vi "PrefDialog.vi"(8 "error in (no error)":errorcluster, 11 "ChromaPowerSupplyModel in":refnum<class "ChromaPowerSupplyModel.lvclass">) -> (0 "error out":errorcluster, 1 "Save As":bool, 2 "Changed":bool, 3 "MyPluginsBase out":refnum<class "ChromaPowerSupplyModel.lvclass">)   [LabVIEW 2018, in "AcPwrPlugins.lvlib" / "ChromaPowerSupplyModel.lvclass"]
doc: "This VI displays the prior instruments properties and allows a user to change the instrument properties and save these new set properties to the same location on disk or in a new location with a new name called \"Type\"."
uses:
  ChromaPowerSupplyModel.lvclass
  C:/Program Files (x86)/National Instruments/LabVIEW 2018/user.lib/NIST/BaseClasses/BasePlugin_class/BasePlugin.lvclass
  C:/Projects/SmartGrid/ICDAS/NistPluggableModules/AcPwr/AcPwrPlugins/AcPwrBaseClass/AcPwrBase.lvclass
  ChromaPowerSupplyClass/TypeDefs/Measurements.ctl
  AcPwrBaseClass/TypeDefs/BaseMeasurements.ctl
  ChromaAcLoadClass/TypeDefs/MeasurementType.ctl
  ChromaPowerSupplyClass/TypeDefs/Device(s)Settings.ctl
  TypeDefs/Database Settings.ctl
  <userlib>/NIST/BaseClasses/BasePlugin_class/BasePlugin.lvclass/BasePlugin.ctl
  AcPwrBaseClass/AcPwrBase.lvclass/AcPwrBase.ctl
  <userlib>/NIST/BaseClasses/BasePlugin_class/Accessors/Read PluginIniFilePath.vi
  AcPwrBaseClass/Accessors/Read BaseConfig.vi
  AcPwrBaseClass/Accessors/Read BaseMeasurements.vi
  <userlib>/NIST/BaseClasses/BasePlugin_class/Accessors/Write PluginIniFilePath.vi
  <vilib>/Utility/config.llb/NI_LVConfig.lvlib
  AcPwrBaseClass/AcPwrBase.lvclass
  ChromaPowerSupplyClass/ChromaPowerSupply.lvclass
  ChromaAcLoadClass/ChromaAcLoad.lvclass
panel:
  in  "Database Settings":T1
  in  "btnSaveAs":bool
  in  "btnSave":bool
  in  "Measurement RefreshTime (ms)":u32
  in  "Device(s)Settings":T2
  in  "BaseMeasurements":T3 {"NHRGridSim Phase" items=["All", "A Phase", "B Phase", "C Phase"]; "NHRDC Measurement Type" items=["Voltage"=1, "Positive Peak Voltage"=2, "Positive Peak Voltage Last Fetch"=4, "Negative Peak Voltage"=8, "Negative Peak Voltage Last Fetch"=16, "Current"=32, "Positive Peak Current"=64, "Positive Peak Current Last Fetch"=128, "Negative Peak Current"=256, "Negative Peak Current Last Fetch"=512, "Power"=1024, "Positive Peak Power"=2048, "Positive Peak Power Last Fetch"=4096, "Negative Peak Power"=8192, "Negative Peak Power Last Fetch"=16384, "Timestamp"=32768, "Charge Time"=65536, "Discharge Time"=131072, "Amp Hour"=262144, "Amp Hour Time"=524288, "Amp Hour Charge"=1048576, "Amp Hour Discharge"=2097152, "Kilo Watt Hour"=4194304, "Kilo Watt Hour Time"=8388608, "Kilo Watt Hour Charge"=16777216, "Kilo Watt Hour Discharge"=33554432, "UUT Temperature"=67108864]; "NHRDC Fetch Method" items=["Aperture", "Immediate"]}
  in  "Measurements":T5
  in  "btnCancel":bool
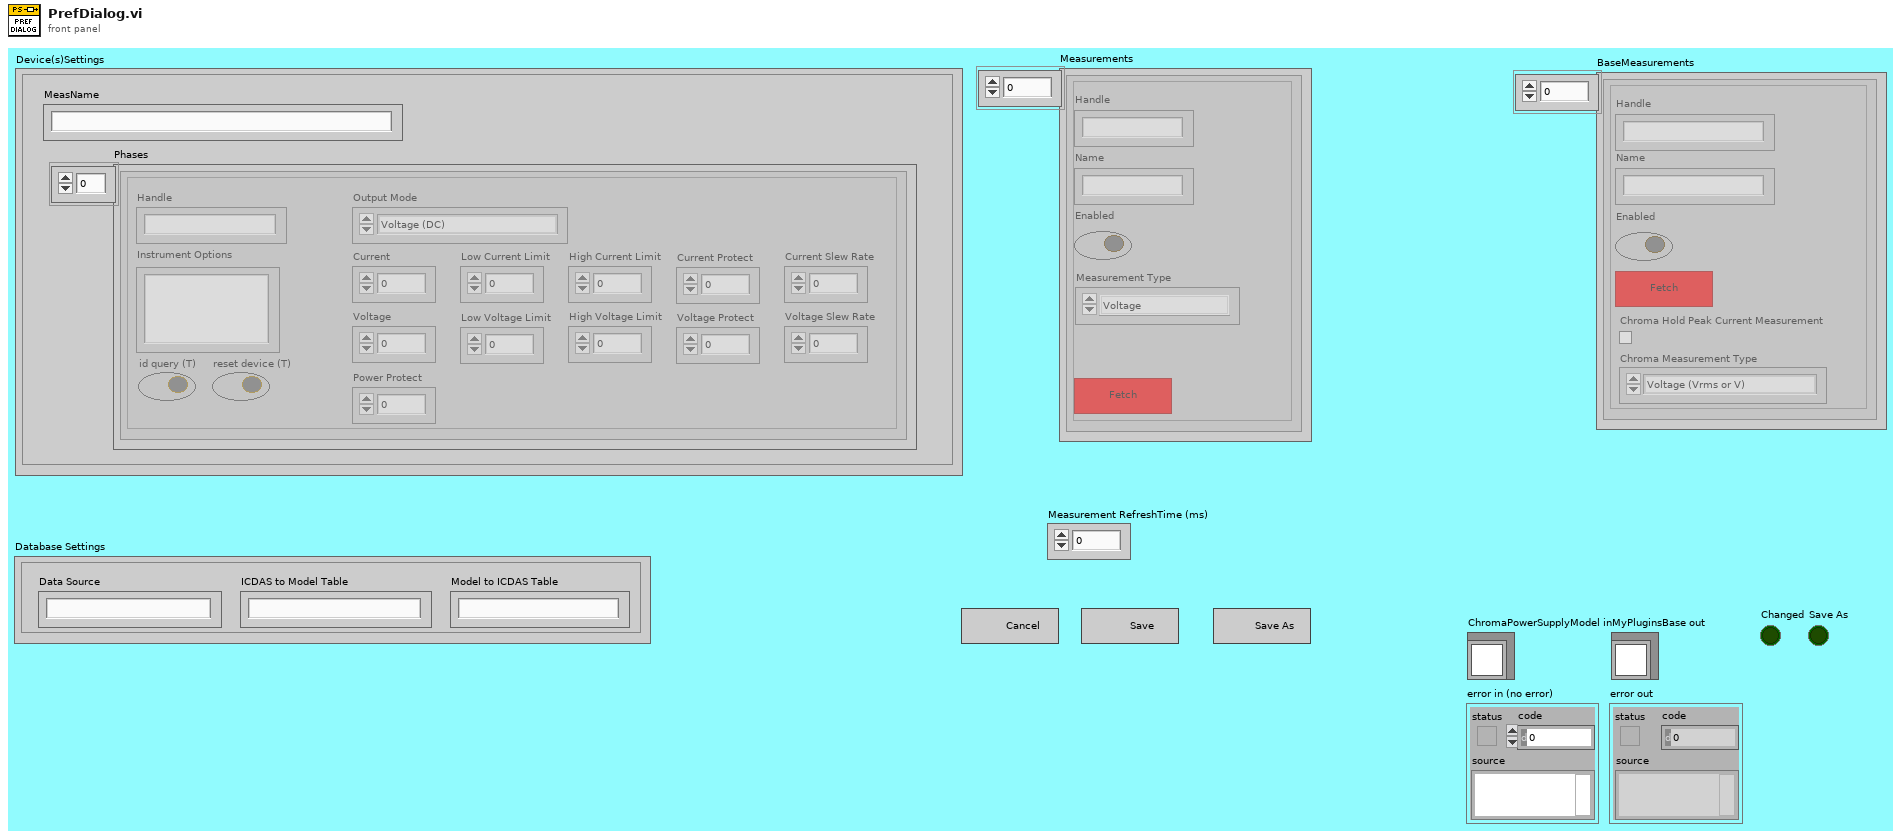
[diagram p1: front panel]
types:
  T1 = typedef "AcPwrPlugins.lvlib/ChromaPowerSupplyModel.lvclass/Database Settings.ctl" = cluster{"Data Source":string, "ICDAS to Model Table":string, "Model to ICDAS Table":string}
  T2 = typedef "AcPwrPlugins.lvlib/ChromaPowerSupply.lvclass/Device(s)Settings.ctl" = cluster{"Phases":cluster{"Handle":string, "Instrument Options":string, "id query (T)":bool, "reset device (T)":bool, "Timing":cluster{"TimingOn":enum16{""}, "Hours":u32, "Minutes":u32, "Seconds":dbl, "CutoffVoltage":dbl}, "Connected":bool, "Output Mode":enum16{"Voltage (DC)", "Current (DC)"}, "Voltage":dbl, "Current":dbl, "High Voltage Limit":dbl, "High Current Limit":dbl, "Power Protect":dbl, "Current Protect":dbl, "Voltage Protect":dbl, "Low Current Limit":dbl, "Low Voltage Limit":dbl, "Current Slew Rate":dbl, "Voltage Slew Rate":dbl}[], "MeasName":string}
  T3 = typedef "AcPwrPlugins.lvlib/AcPwrBase.lvclass/BaseMeasurements.ctl" = cluster{"Handle":string, "Name":string, "Enabled":bool, "Measurement Value":dbl, "btnMeasFetch":bool, "Chroma Hold Peak Current Measurement":bool, "Chroma Measurement Type":T4, "Chroma Protection Status String":string, "NHRDC Fetch Method":i32, "NHRDC Fetch Time (s)":sgl, "NHRDC Measurement Type":i32, "NHRGridSim Measurement Type ":enum16{"Average Current", "Max Current", "Min Current", "Average Voltage", "Max Voltage", "Min Voltage", "Average True Power", "Max True Power", "Min True Power", "Average Apparent Power", "Max Apparent Power", "Min Apparent Power", "Power Factor", "Crest Factor"}, "NHRGridSim Phase ":i32, "PPS Measurement Type ":enum16{"Voltage RMS L-N", "Voltage RMS L-L", "Frequency", "Current RMS", "Current Peak", "Crest Factor", "Power Factor", "Power VA", "Real Power"}, "PPS Channel Name":enum16{"A", "B", "C"}}[]
  T4 = typedef "AcPwrPlugins.lvlib/ChromaAcLoad.lvclass/MeasurementType.ctl" = enum16{"Voltage (Vrms or V)", "Current (Arms or A)", "Power (W)", "Peak Voltage (V)", "Peak Current (A)", "Peak Power (W)", "Frequency (Hz)", "Resistance (Ohms)", "Voltage Overshoot (V)", "Positive Peak Current (A)", "Voltage Undershoot (V)", "Negative Peak Current (A)", "Apparent Power (VA)", "Reacitive Power (VAR)", "Voltage THD", "Power Factor", "Current's Crest Factor"}
  T5 = typedef "AcPwrPlugins.lvlib/ChromaPowerSupply.lvclass/Measurements.ctl" = cluster{"Handle":string, "Name":string, "Enabled":bool, "Measurement Value":dbl, "btnMeasFetch":bool, "ProtectionStatusString":string, "Measurement Type":enum16{"Voltage", "Current", "Power"}}[]
  T6 = enum32{"Invalid", "Default", "Floating", "Floating/Auto-Hide", "Modal"}
  T7 = enum32{"Invalid", "Standard", "Closed", "Hidden", "Minimized", "Maximized"}
  T8 = enum8{"Enabled", "Disabled", "Disabled and Grayed Out"}
  T9 = cluster{"Handle":string, "Instrument Options":string, "id query (T)":bool, "reset device (T)":bool, "Timing":cluster{"TimingOn":enum16{""}, "Hours":u32, "Minutes":u32, "Seconds":dbl, "CutoffVoltage":dbl}, "Connected":bool, "Output Mode":enum16{"Voltage (DC)", "Current (DC)"}, "Voltage":dbl, "Current":dbl, "High Voltage Limit":dbl, "High Current Limit":dbl, "Power Protect":dbl, "Current Protect":dbl, "Voltage Protect":dbl, "Low Current Limit":dbl, "Low Voltage Limit":dbl, "Current Slew Rate":dbl, "Voltage Slew Rate":dbl}[]
  T10 = cluster{"Device(s)Settings":T2, "Database Settings":T1}
  T11 = cluster{"Handle":string, "Instrument Options":string, "id query (T)":bool, "reset device (T)":bool, "Timing":cluster{"TimingOn":enum16{""}, "Hours":u32, "Minutes":u32, "Seconds":dbl, "CutoffVoltage":dbl}, "Connected":bool, "Output Mode":enum16{"Voltage (DC)", "Current (DC)"}, "Voltage":dbl, "Current":dbl, "High Voltage Limit":dbl, "High Current Limit":dbl, "Power Protect":dbl, "Current Protect":dbl, "Voltage Protect":dbl, "Low Current Limit":dbl, "Low Voltage Limit":dbl, "Current Slew Rate":dbl, "Voltage Slew Rate":dbl}
  T12 = typedef "AcPwrPlugins.lvlib/AcPwrBase.lvclass/BaseConfig.ctl" = cluster{"Frequency":dbl, "FrequencyRange":dbl[], "Phases":T13[], "Name":string, "PluginConfigVariant":variant, "PluginMeasVariant":variant}
  T13 = typedef "AcPwrPlugins.lvlib/AcPwrBase.lvclass/Phase.ctl" = cluster{"Name":string, "Enabled":bool, "VoltageLevel":dbl, "Handle":string, "VoltageRange":dbl[], "Connected":bool, "CurrentLimit":dbl, "Waveform":string}
  T14 = typedef "NI_LVConfig.lvlib/Config Data RefNum.ctl" = refnum<k1>
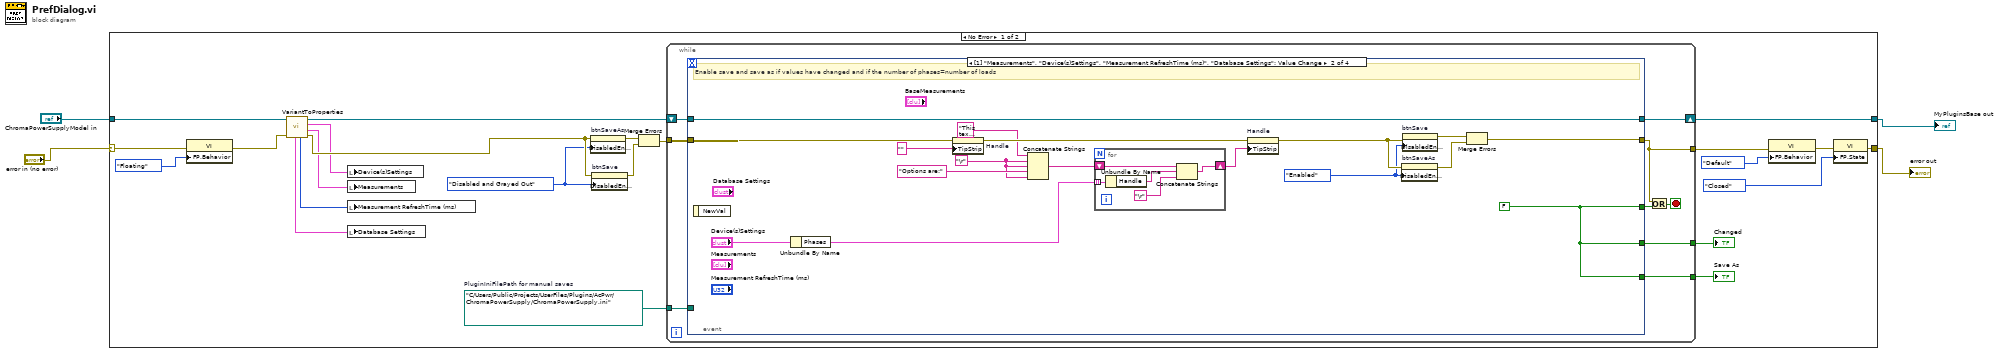
[diagram p0: block diagram]
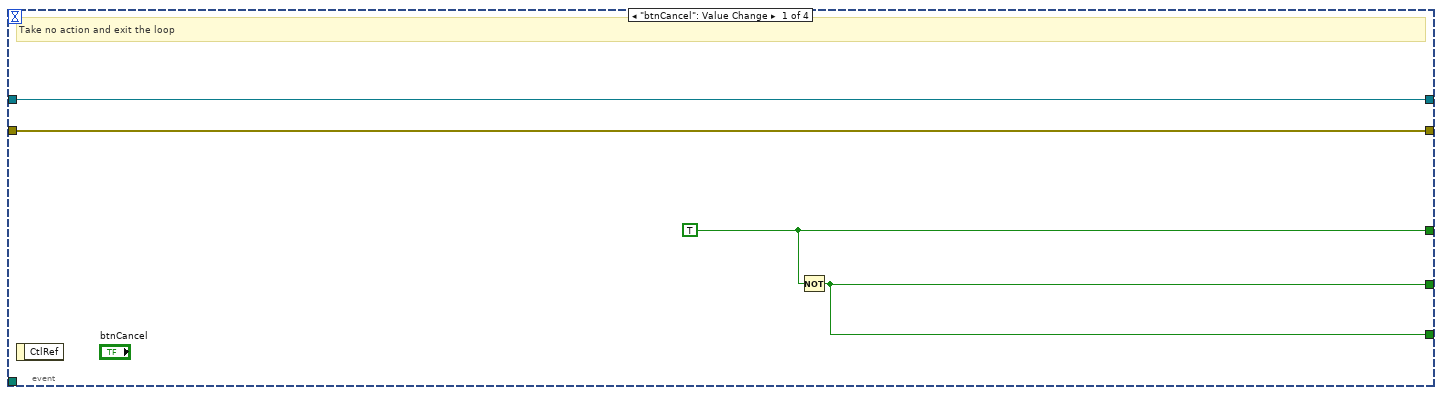
[diagram p2: hidden frame]
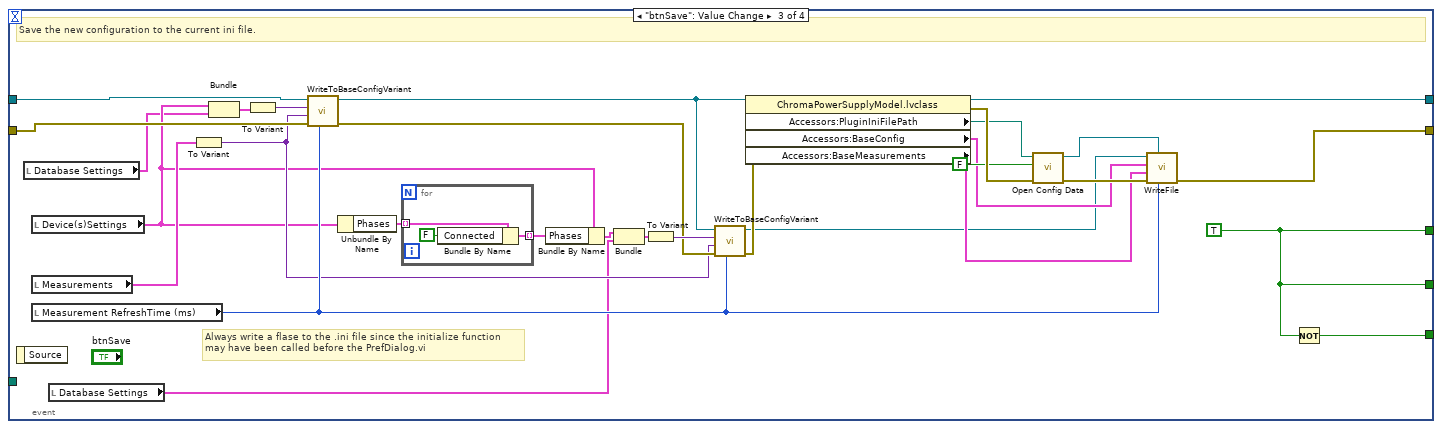
[diagram p3: hidden frame]
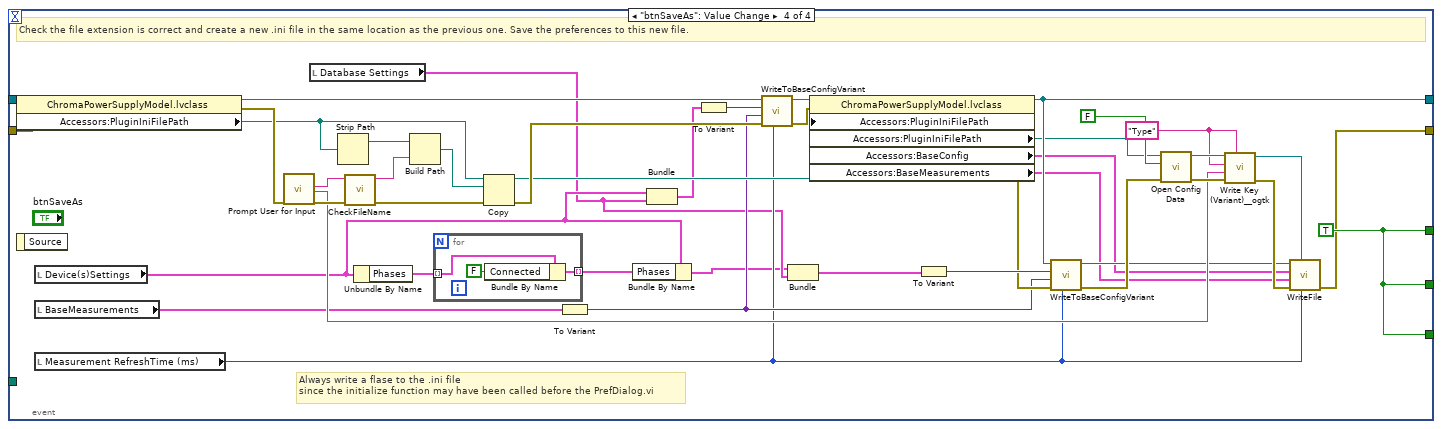
[diagram p4: hidden frame]
diagram:
  n1 = case shown="No Error" "error in (no error)" {
    selector: "error in (no error)" -> [w20 w142]
    tunnel: [w27 w143] -> w2
    tunnel: [w23 w142] -> w1
    tunnel: "ChromaPowerSupplyModel in" -> [w22 w143]
    frame No Error {
      w12 = T8."Disabled and Grayed Out" ("Disabled")
      w8 = path "C:/Users/Public/Projects/UserFiles/Plugins/AcPwr/ChromaPowerSupply/ChromaPowerSupply.ini"  # PluginIniFilePath for manual saves
      n2 = property class="VI"(error in=w20, "FP.Behavior"=T6."Floating" ("Front Panel Window:Behavior")) -> (error out=w18:errorcluster)  [unwired: 1 in, 1 out]
      n3 = call "VariantToProperties.vi"("error in (no error)"=w18, "ChromaPowerSupplyModel in"=w22) -> ("error out"=w16:errorcluster, "Measurements"=w9:T5, "Device Settings"=w11:T2, "ChromaPowerSupplyModel out"=w15:refnum<class "ChromaPowerSupplyModel.lvclass">, "Measurement Refresh Time (ms)"=w10:u32, "Database Settings"=w5:T1)  [unwired: 4 in]
      n4 = local write "Device(s)Settings"(w11) -> ()
      n5 = local write "Measurements"(w9) -> ()
      n6 = local write "Measurement RefreshTime (ms)"(w10) -> ()
      n7 = local write "Database Settings"(w5) -> ()
      n8 = property on="btnSaveAs" class="Bool"(error in=w16, "DisabledEnum"=w12) -> (error out=w13:errorcluster)  [unwired: 1 in, 1 out]
      n9 = property on="btnSave" class="Bool"(error in=w16, "DisabledEnum"=w12) -> (error out=w14:errorcluster)  [unwired: 1 in, 1 out]
      n10 = Merge Errors(w13, w14) -> (w17:errorcluster)
      n11 = while {
        shift-right: [w35] -> w27
        shift-left: w15 -> [w36]
        tunnel: w17 -> [w34]
        tunnel: [w30] -> w21
        tunnel: [w33] -> w7
        tunnel: [w32] -> w6
        tunnel: w8 -> [w28]
        stop <- w31 stop-if-true
        n12 = event shown="[1] \"Measurements\", \"Device(s)Settings\", \"Measurement RefreshTime (ms)\", \"Database Settings\": Value Change" {
          selector: _ -> [_ _ _ _]
          dyn-events: _ -> [_ _ _ _]
          timeout: _ -> [_ _ _ _]
          tunnel: w36 -> [w40 w55 w69 w126]
          tunnel: [w38 w56 w90 w132] -> w29
          tunnel: [w40 w55 w77 w108] -> w35
          tunnel: w34 -> [w39 w51 w83 w125]
          tunnel: [w39 w57 w84 w119] -> w30
          tunnel: [w37 w56 w90 w132] -> w33
          tunnel: [w37 w56 w89 w132] -> w32
          tunnel: w28 -> [_ _ _ _]
          event "btnCancel": Value Change {
            w38 = TRUE
            # "Take no action and exit the loop"
            n13 = event-data() -> ()  [unwired: 1 in, 1 out]
            n14 = Not(x=w38) -> (.not. x?=w37:bool)
          }
          event "Measurement RefreshTime (ms)": Value Change {
            w41 = T8."Enabled" ("Disabled")
            w47 = "\r"
            w56 = FALSE
            # "Enable save and save as if values have changed and if the number of phases=number of loads"
            n15 = event-data() -> ()  [unwired: 1 in, 1 out]
            n16 = Unbundle By Name("Device(s)Settings") -> ("Phases"=w44:T9)
            n17 = property on="Handle" class="Str"(error in=w51, "TipStrip"="" ("Tip Strip")) -> (error out=w53:errorcluster)  [unwired: 1 in, 1 out]
            n18 = Concatenate Strings("This text in this handle of the instrument and entered in the  \nhandle control in the Phases array EXACTLY, lest the attempt \nto interact with the instrument will fail.", w47, w47, "Options are:" ("Handle"), w47) -> (w52:string)
            n19 = for {
              shift-right: [w62] -> w54
              shift-left: w52 -> [w61]
              tunnel: w44 -> [w60] mode=indexing
              n20 = Unbundle By Name(w60) -> ("Handle"=w59:string)
              n21 = Concatenate Strings(w61, w59, "\r") -> (w62:string)
            }
            n22 = property on="Handle" class="Str"(error in=w53, "TipStrip"=w54) -> (error out=w45:errorcluster)  [unwired: 1 in, 1 out]
            n23 = property on="btnSaveAs" class="Bool"(error in=w45, "DisabledEnum"=w41) -> (error out=w43:errorcluster)  [unwired: 1 in, 1 out]
            n24 = property on="btnSave" class="Bool"(error in=w45, "DisabledEnum"=w41) -> (error out=w42:errorcluster)  [unwired: 1 in, 1 out]
            n25 = Merge Errors(w42, w43) -> (w57:errorcluster)
          }
          event "btnSave": Value Change {
            w90 = TRUE
            # "Always write a flase to the .ini file since the initialize function\nmay have been called before the PrefDialog.vi"
            # "Save the new configuration to the current ini file."
            n26 = event-data() -> ()  [unwired: 1 in, 1 out]
            n27 = local read "Database Settings"() -> (w63:T1)
            n28 = local read "Device(s)Settings"() -> (w64:T2)
            n29 = local read "Measurements"() -> (w73:T5)
            n30 = local read "Measurement RefreshTime (ms)"() -> (w75:u32)
            n31 = local read "Database Settings"() -> (w66:T1)
            n32 = To Variant(anything=w73) -> (Variant=w74:variant)
            n33 = Bundle("Device(s)Settings"=w64, "Database Settings"=w63) -> (w65:T10)  [unwired: 1 in]
            n34 = To Variant(anything=w65) -> (Variant=w82:variant)
            n35 = call-dynamic "WriteToBaseConfigVariant.vi"("Measurement Refresh Time (ms)"=w75, "error in (no error)"=w83, "Meas"=w74, "Config"=w82, "ChromaPowerSupplyModel in"=w69) -> ("error out"=w79:errorcluster, "ChromaPowerSupplyModel out"=w80:refnum<class "ChromaPowerSupplyModel.lvclass">)  [unwired: 5 in]
            n36 = Unbundle By Name(w64) -> ("Phases"=w88:T9)
            n37 = for {
              tunnel: w88 -> [w94] mode=indexing
              tunnel: [w95] -> w87 mode=indexing
              n38 = Bundle By Name(cluster=w94, "Connected"=FALSE) -> (w95:T11)
            }
            n39 = Bundle By Name(cluster=w64, "Phases"=w87) -> (w68:T2)
            n40 = Bundle("Device(s)Settings"=w68, "Database Settings"=w66) -> (w67:T10)  [unwired: 1 in]
            n41 = To Variant(anything=w67) -> (Variant=w81:variant)
            n42 = call-dynamic "WriteToBaseConfigVariant.vi"("Measurement Refresh Time (ms)"=w75, "error in (no error)"=w79, "Meas"=w74, "Config"=w81, "ChromaPowerSupplyModel in"=w80) -> ("error out"=w78:errorcluster, "ChromaPowerSupplyModel out"=w70:refnum<class "ChromaPowerSupplyModel.lvclass">)  [unwired: 5 in]
            n43 = property class="ChromaPowerSupplyModel.lvclass"(reference=w80, error in=w78) -> (reference out=w77:refnum<class "ChromaPowerSupplyModel.lvclass">, error out=w92:errorcluster, "Accessors:PluginIniFilePath"=w71:path, "Accessors:BaseConfig"=w76:T12, "Accessors:BaseMeasurements"=w72:T3)
            n44 = call <vilib>:"Open Config Data.vi"("error in (no error)"=w92, "create file if necessary (T)"=FALSE, "configuration file path"=w71) -> ("error out"=w86:errorcluster, "refnum"=w85:T14)  [unwired: 6 in, 1 out]
            n45 = call-dynamic "WriteFile.vi"("RefreshTime"=w75, "Refnum in"=w85, "error in (no error)"=w86, "BaseMeasurements"=w72, "BaseConfiguration"=w76, "MyPluginsBase in"=w70) -> ("error out"=w84:errorcluster)  [unwired: 4 in, 1 out]
            n46 = Not(x=w90) -> (.not. x?=w89:bool)
          }
          event "btnSaveAs": Value Change {
            w133 = "Type" ("section (optional)")
            w132 = TRUE
            # "Always write a flase to the .ini file\nsince the initialize function may have been called before the PrefDialog.vi"
            # "Check the file extension is correct and create a new .ini file in the same location as the previous one. Save the preferences to this new file."
            n47 = property class="ChromaPowerSupplyModel.lvclass"(reference=w126, error in=w125) -> (reference out=w117:refnum<class "ChromaPowerSupplyModel.lvclass">, error out=w124:errorcluster, "Accessors:PluginIniFilePath"=w123:path)
            n48 = event-data() -> ()  [unwired: 1 in, 1 out]
            n49 = local read "Device(s)Settings"() -> (w100:T2)
            n50 = local read "BaseMeasurements"() -> (w103:T3)
            n51 = local read "Measurement RefreshTime (ms)"() -> (w101:u32)
            n52 = call "Prompt User for Input"("error in (no error)"=w124) -> ("File Name"=w127:string, "PluginType"=w130:string, "error out"=w131:errorcluster)  [unwired: 15 in, 1 out]
            n53 = local read "Database Settings"() -> (w98:T1)
            n54 = Strip Path(path=w123) -> (stripped path=w137:path)  [unwired: 1 out]
            n55 = call "CheckFileName.vi"("Error In"=w131, "File Name in"=w127) -> ("Error Out"=w129:errorcluster, "File Name out"=w128:string)  [unwired: 8 in]
            n56 = Unbundle By Name(w100) -> ("Phases"=w122:T9)
            n57 = Build Path(base path=w137, name or relative path=w128) -> (appended path=w136:path)
            n58 = for {
              tunnel: w122 -> [w139] mode=indexing
              tunnel: [w141] -> w121 mode=indexing
              n59 = Bundle By Name(cluster=w139, "Connected"=FALSE) -> (w141:T11)
            }
            n60 = Copy(8:w129, 10:w136, 11:w123) -> (0:w115:errorcluster, 3:w107:path)  [unwired: 2 in, 1 out]
            n61 = To Variant(anything=w103) -> (Variant=w102:variant)
            n62 = Bundle By Name(cluster=w100, "Phases"=w121) -> (w97:T2)
            n63 = Bundle("Device(s)Settings"=w100, "Database Settings"=w98) -> (w99:T10)  [unwired: 1 in]
            n64 = To Variant(anything=w99) -> (Variant=w114:variant)
            n65 = call-dynamic "WriteToBaseConfigVariant.vi"("Measurement Refresh Time (ms)"=w101, "error in (no error)"=w115, "Meas"=w102, "Config"=w114, "ChromaPowerSupplyModel in"=w117) -> ("error out"=w116:errorcluster, "ChromaPowerSupplyModel out"=w112:refnum<class "ChromaPowerSupplyModel.lvclass">)  [unwired: 5 in]
            n66 = Bundle("Device(s)Settings"=w97, "Database Settings"=w98) -> (w96:T10)  [unwired: 1 in]
            n67 = property class="ChromaPowerSupplyModel.lvclass"(reference=w112, error in=w116, "Accessors:PluginIniFilePath"=w107) -> (reference out=w108:refnum<class "ChromaPowerSupplyModel.lvclass">, error out=w111:errorcluster, "Accessors:PluginIniFilePath"=w106:path, "Accessors:BaseConfig"=w105:T12, "Accessors:BaseMeasurements"=w104:T3)
            n68 = To Variant(anything=w96) -> (Variant=w113:variant)
            n69 = call-dynamic "WriteToBaseConfigVariant.vi"("Measurement Refresh Time (ms)"=w101, "error in (no error)"=w111, "Meas"=w102, "Config"=w113, "ChromaPowerSupplyModel in"=w108) -> ("error out"=w110:errorcluster, "ChromaPowerSupplyModel out"=w109:refnum<class "ChromaPowerSupplyModel.lvclass">)  [unwired: 5 in]
            n70 = call <vilib>:"Open Config Data.vi"("error in (no error)"=w110, "create file if necessary (T)"=FALSE, "configuration file path"=w106) -> ("error out"=w135:errorcluster, "refnum"=w134:T14)  [unwired: 6 in, 1 out]
            n71 = call <userlib>:"Write Key (Variant)__ogtk.vi"("section"=w133, "error in (no error)"=w135, "key-value"=w130, "key (optional)"=w133, "refnum"=w134) -> ("error out"=w120:errorcluster, "refnum out"=w118:T14)  [unwired: 5 in]
            n72 = call-dynamic "WriteFile.vi"("RefreshTime"=w101, "Refnum in"=w118, "error in (no error)"=w120, "BaseMeasurements"=w104, "BaseConfiguration"=w105, "MyPluginsBase in"=w109) -> ("error out"=w119:errorcluster)  [unwired: 4 in, 1 out]
          }
        }
        n73 = Or(x=w30, y=w29) -> (x .or. y?=w31:bool)
      }
      "Save As" <- w6
      "Changed" <- w7
      n74 = property class="VI"(error in=w21, "FP.Behavior"=T6."Default" ("Front Panel Window:Behavior")) -> (error out=w26:errorcluster)  [unwired: 1 in, 1 out]
      n75 = property class="VI"(error in=w26, "FP.State"=T7."Closed" ("Front Panel Window:State")) -> (error out=w23:errorcluster)  [unwired: 1 in, 1 out]
    }
    frame Error {
    }
  }
  "error out" <- w1
  "MyPluginsBase out" <- w2
